vi "Main.vi"() -> ()   [LabVIEW 2026]
doc: "This template is for the Queued Message Handler design pattern.\n\nThe Event Handling Loop generates messages based on user interface actions.\n\nThe Message Handling Loop processes messages generated by the Event Handling Loop, or by other messages. The messages are string values, so new messages can be added easily to the Message Cases case structure in the Message Handling Loop. Each message cluster can also provide an optional value for Message Data, which is a variant that can be converted to whatever message-specific data is required."
uses:
  Controls/Telemetry_Data_Type.ctl
  Controls/Channels.ctl
  Acquisition/Controls/Alarms.ctl
  Controls/UI_Data_Type.ctl
  Controls/Waveforms.ctl
  Controls/UI State.ctl
  Support/Message Queue/Enqueue Message (Single).vi
  <vilib>/Utility/error.llb/Error Cluster From Error Code.vi
  <vilib>/ErrorRing/Error Ring.xnode
  support/Message Queue/Message Queue.lvlib
  support/User Event - Stop/User Event - Stop.lvlib
  Acquisition/Acquisition.lvlib
  TCP/TCP.lvlib
  Database/Database.lvlib
  Data Logging/Data Logging.lvlib
  <vilib>/Analysis/NI_AALPro.lvlib
panel:
  out "Alarms":T1
  out "Telemetry Data":T2
  out "Vibration Frequency Spectrum":waveform(dbl)[](graph)
  out "Vibration Display":waveform(dbl)[](graph)
  in  "Start Acquisition":bool
  out "Display":string
  in  "Exit":bool
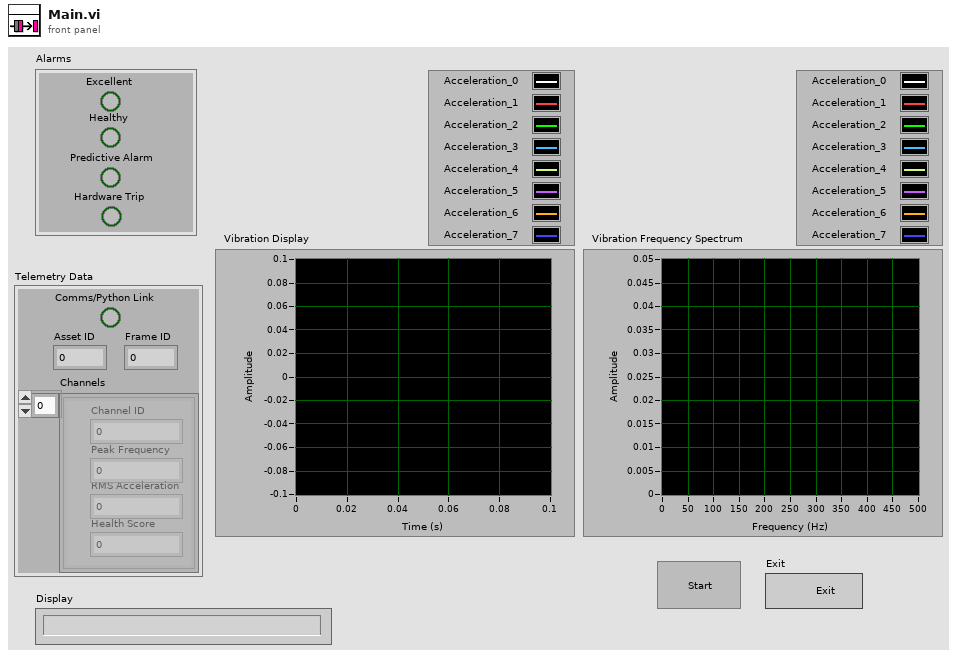
[diagram p1: front panel]
types:
  T1 = typedef "Acquisition.lvlib/Alarms.ctl" = cluster{"Excellent":bool, "Healthy":bool, "Predictive Alarm":bool, "Hardware Trip":bool}
  T2 = typedef "Telemetry_Data_Type.ctl" = cluster{"asset_id":i32, "frame_id":i32, "channels":T3, "comms/python link":bool}
  T3 = typedef "Channels.ctl" = cluster{"channel_id":dbl, "peak_frequency":dbl, "rms_acceleration":dbl, "health_score":dbl}[]
  T4 = typedef "UI State.ctl" = enum16{"Idle", "Acquiring and Logging", "Waiting for Exit", "Waiting for Exit (Acq Stopped)", "Waiting for Exit (Log Stopped)", "Waiting for Stop", "Waiting for Stop (Acq Stopped)", "Waiting for Stop (Log Stopped)"}
  T5 = typedef "Waveforms.ctl" = waveform(dbl)[]
  T6 = typedef "UI_Data_Type.ctl" = cluster{"Boolean":bool, "String":string, "Numeric ":dbl, "Data Display Ref":refnum<vi>, "Exit Button Ref":refnum<vi>}
  T7 = typedef "Message Queue.lvlib/All Message Queues.ctl" = cluster{"UI":refnum<queue>, "Database":refnum<queue>, "TCP":refnum<queue>, "Acquisition":refnum<queue>, "Data Logging":refnum<queue>}
  T8 = typedef "Vibration_Monitor_Config.ctl" = cluster{"Diagnostic_Modes":cluster{"Selected_Mode":string}, "Basic_Health":T9, "Complex_Machinery":T9, "Multi_Point":T9, "System_Settings":T10}
  T9 = typedef "Vibration_Profile.ctl" = cluster{"Task_Name":string, "Sample_Rate_Hz":dbl, "Samples_Per_Channel":i32}
  T10 = typedef "System_Settings.ctl" = cluster{"Simulation_Mode ":string, "Options":T11}
  T11 = typedef "Options.ctl" = enum16{"Healthy", "Unbalance_Alert", "Bearing_Fault_Critical", "Sweep_Test"}
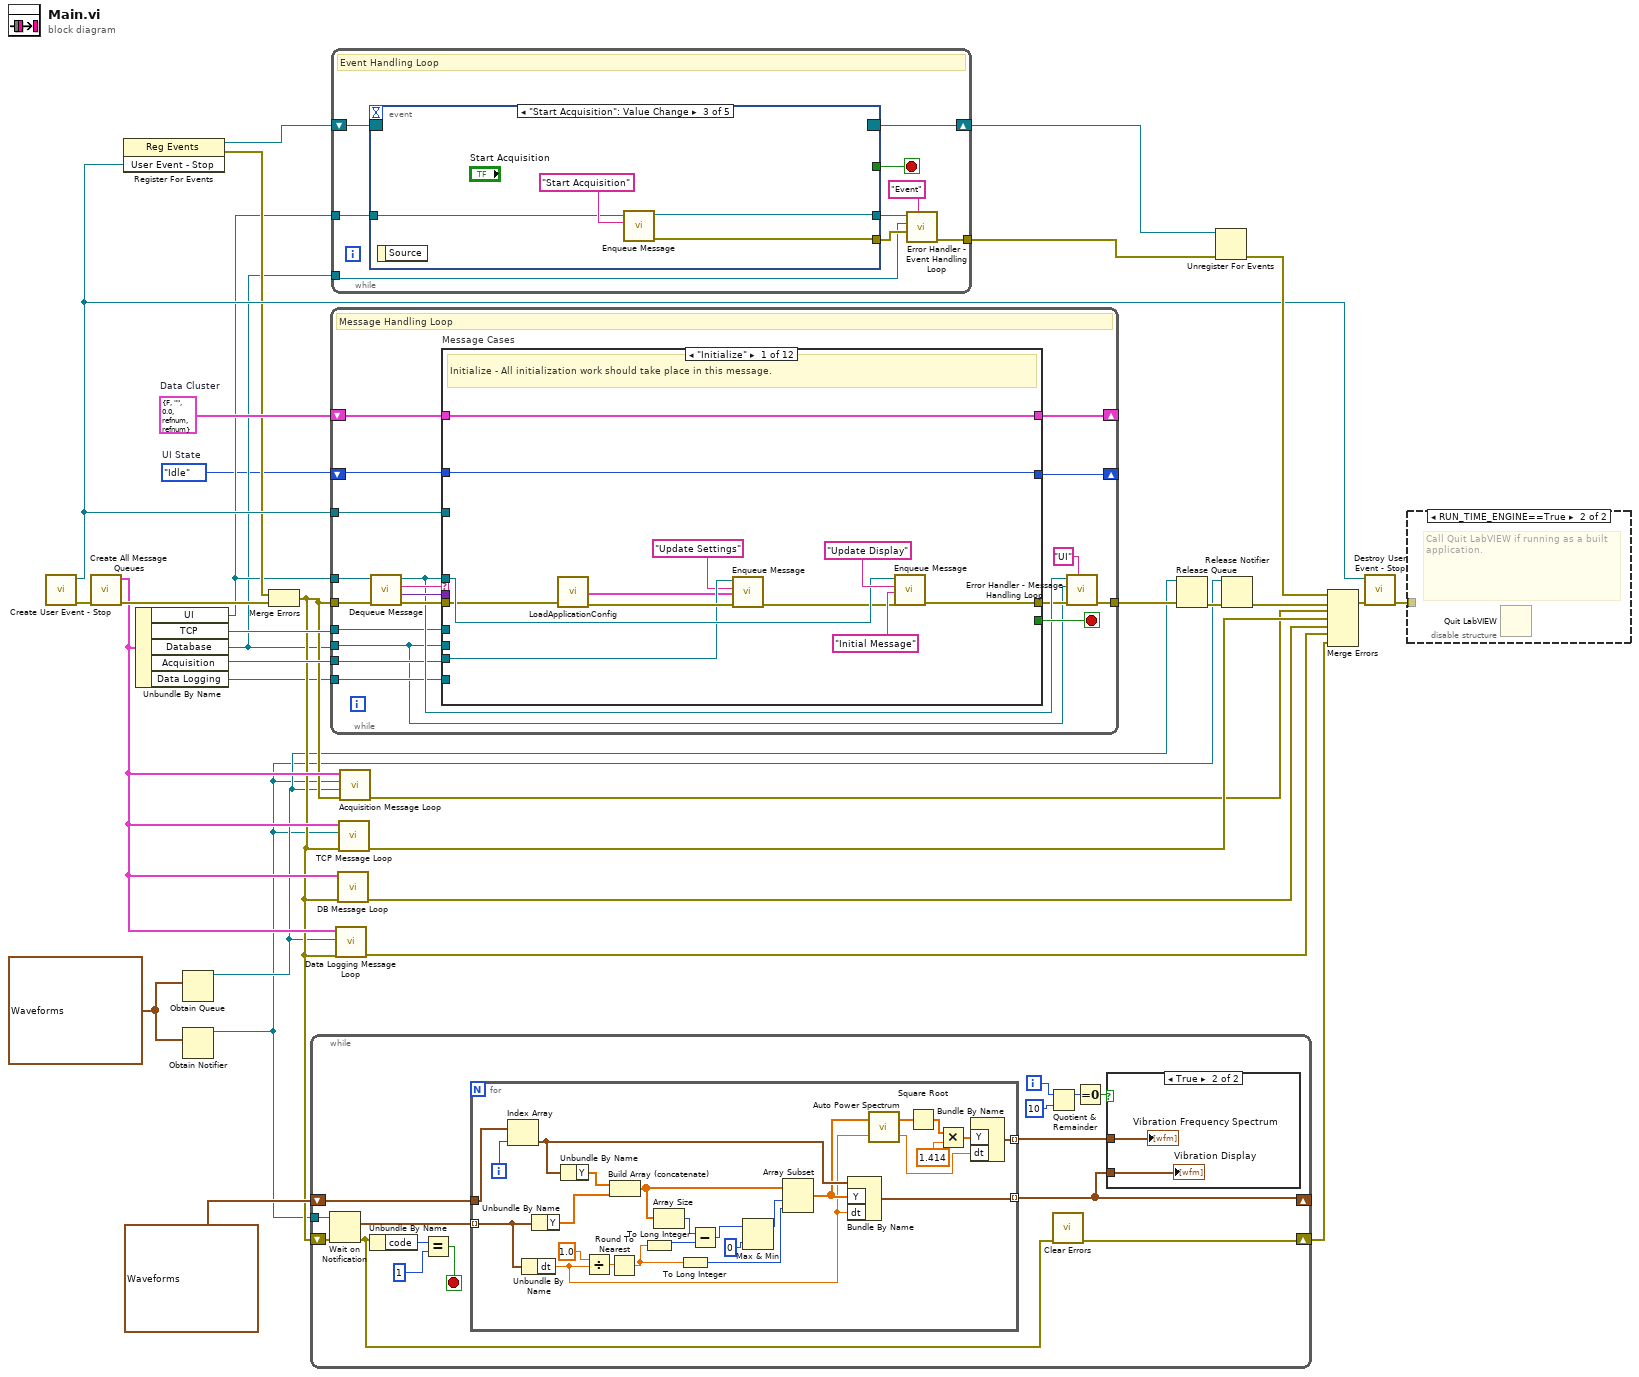
[diagram p0: block diagram]
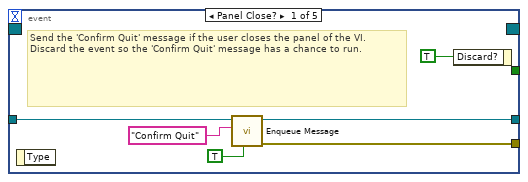
[diagram p4: hidden frame]
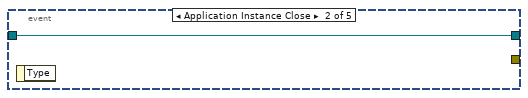
[diagram p5: hidden frame]
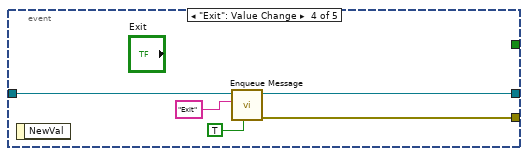
[diagram p6: hidden frame]
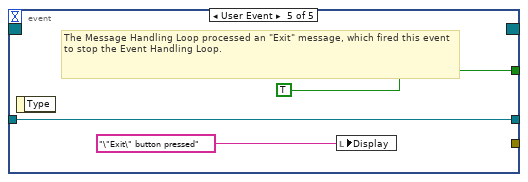
[diagram p7: hidden frame]
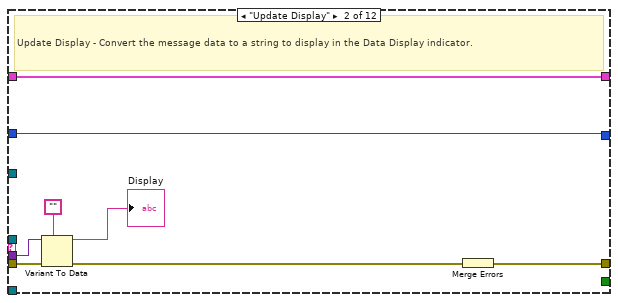
[diagram p8: hidden frame]
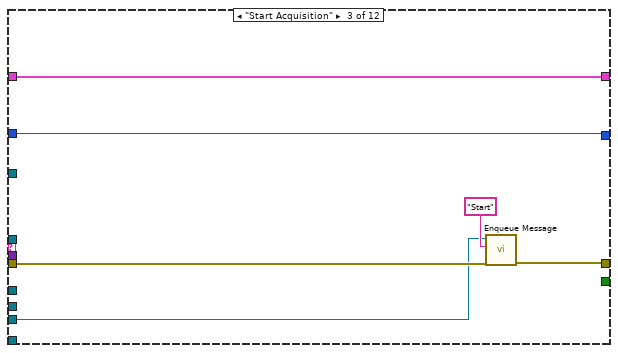
[diagram p9: hidden frame]
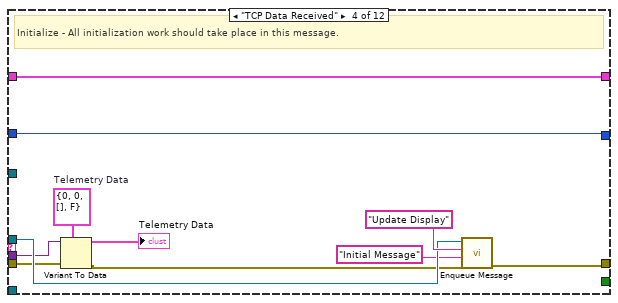
[diagram p10: hidden frame]
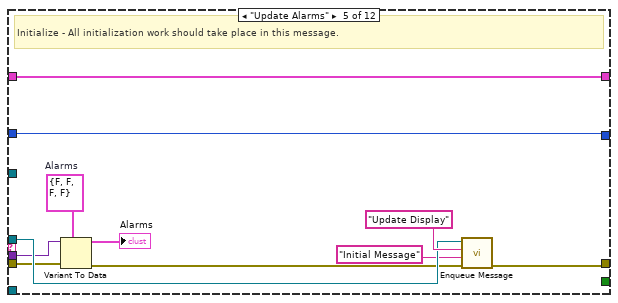
[diagram p11: hidden frame]
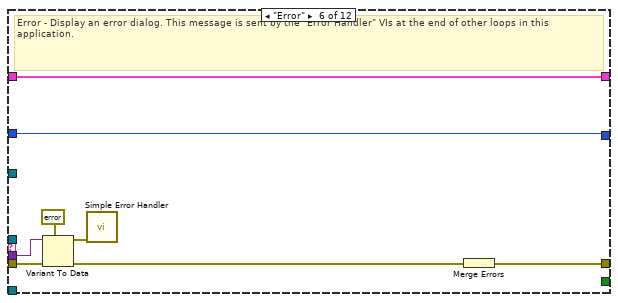
[diagram p12: hidden frame]
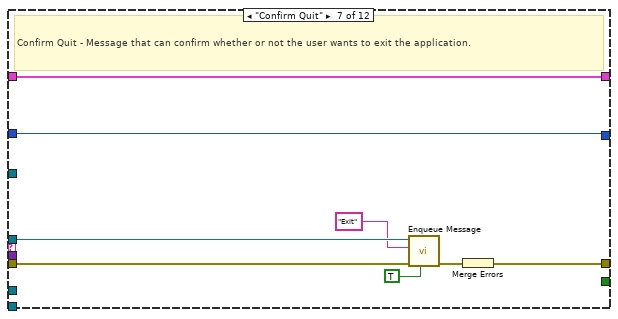
[diagram p13: hidden frame]
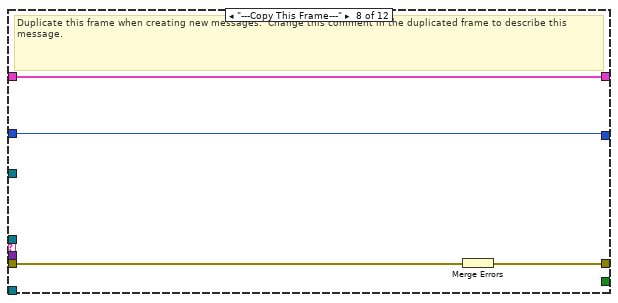
[diagram p14: hidden frame]
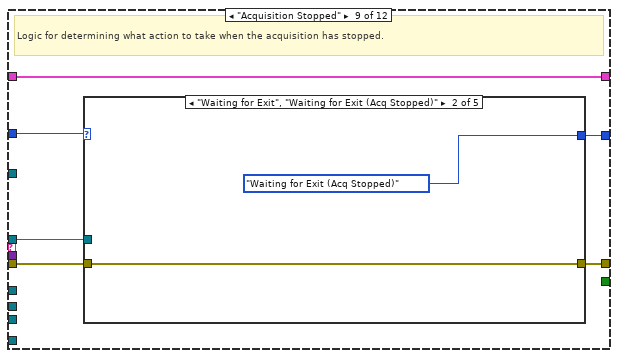
[diagram p15: hidden frame]
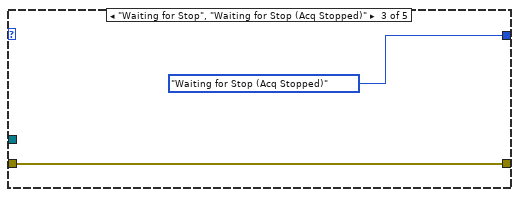
[diagram p17: hidden frame]
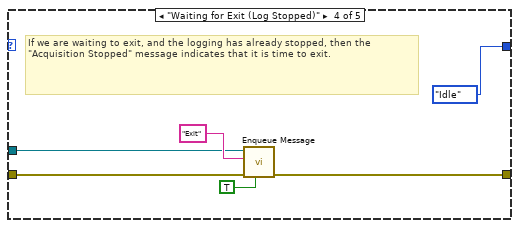
[diagram p18: hidden frame]
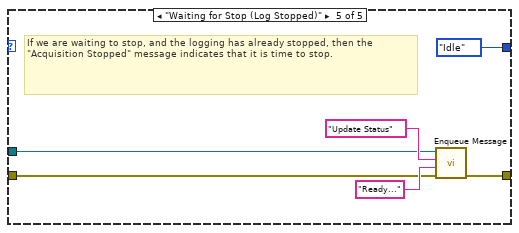
[diagram p19: hidden frame]
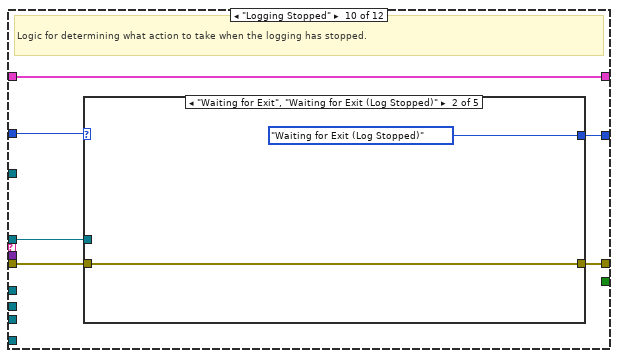
[diagram p20: hidden frame]
diagram:
  w1 = UI_State."Idle"  # UI State
  w17 = T5 [{"t0"=timestamp(0 s since 1904-01-01), "dt"=1.0, "Y"=[0.0]}]
  w26 = T6 {"Boolean"=FALSE, "String"="", "Numeric "=0.0, "Data Display Ref"=refnum, "Exit Button Ref"=refnum}  # Data Cluster
  n1 = call "Create User Event - Stop.vi"() -> ("error out"=w30:errorcluster, "User Event - Stop"=w22:refnum<user-event>)  [unwired: 10 in]
  n2 = call "Create All Message Queues.vi"("error in (no error)"=w30) -> ("error out"=w31:errorcluster, "Message Queues out"=w9:T7)  [unwired: 9 in]
  n3 = register-events(w22) -> (reference out=w23:refnum<event-registration>, error out=w21:errorcluster)  [unwired: 2 in]
  n4 = Unbundle By Name(w9) -> ("UI"=w18:refnum<queue>, "TCP"=w19:refnum<queue>, "Database"=w2:refnum<queue>, "Acquisition"=w11:refnum<queue>, "Data Logging"=w5:refnum<queue>)
  n5 = Obtain Queue(element data type=w17) -> (queue out=w4:refnum<queue>)  [unwired: 4 in, 2 out]
  n6 = Obtain Notifier(notification data type=w17) -> (notifier out=w3:refnum<notifier>)  [unwired: 3 in, 2 out]
  n7 = Merge Errors(w21, w31) -> (w8:errorcluster)
  n8 = while {
    tunnel: w3 -> [w46]
    shift-right: [w39] -> _
    shift-left: T5 [{"t0"=timestamp(0 s since 1904-01-01), "dt"=1.0, "Y"=[0.0]}] ("Waveform") -> [w40]
    shift-right: [w37] -> w7
    shift-left: w8 -> [w45]
    i -> [w36]
    stop <- w44 stop-if-true
    n9 = Wait on Notification(notifier=w46, error in (no error)=w45) -> (notification=w41:T5, error out=w38:errorcluster)  [unwired: 2 in, 2 out]
    n10 = Unbundle By Name(w38) -> ("code"=w43:i32)
    n11 = Equal?(x=w43, y=1) -> (x = y?=w44:bool)
    n12 = for {
      tunnel: w41 -> [w62] mode=indexing
      tunnel: w40 -> [w65]
      tunnel: [w58] -> w39 mode=indexing
      tunnel: [w52] -> w32 mode=indexing
      i -> [w57]
      n13 = Index Array(array=w65, index=w57) -> (element=w63:waveform(dbl))
      n14 = Unbundle By Name(w62) -> ("dt"=w53:dbl)
      n15 = Unbundle By Name(w62) -> ("Y"=w72:dbl[])
      n16 = Unbundle By Name(w63) -> ("Y"=w64:dbl[])
      n17 = Divide(x=1.0, y=w53) -> (x/y=w71:dbl)
      n18 = Round To Nearest(number=w71) -> (nearest integer value=w67:dbl)
      n19 = Build Array (concatenate)(w64, w72) -> (w70:dbl[])
      n20 = To Long Integer(number=w67) -> (32bit integer=w68:i32)
      n21 = Array Size(array=w70) -> (size(s)=w69:i32)
      n22 = To Long Integer(number=w67) -> (32bit integer=w66:i32)
      n23 = Subtract(x=w69, y=w68) -> (x-y=w61:i32)
      n24 = Max & Min(x=w61, y=0) -> (max(x,y)=w59:i32)  [unwired: 1 out]
      n25 = Array Subset(array=w70, index=w59, length=w66) -> (w56:dbl[])
      n26 = Bundle By Name(cluster=w63, "Y"=w56, "dt"=w53) -> (w58:waveform(dbl))
      n27 = call <vilib>:"Auto Power Spectrum.vi"("dt"=w53, "Signal (V)"=w56) -> ("df"=w51:dbl, "Power Spectrum (V^2 rms)"=w50:dbl[])
      n28 = Square Root(x=w50) -> (sqrt(x)=w49:dbl[])
      n29 = Multiply(x=w49, y=1.414) -> (x*y=w54:dbl[])
      n30 = Bundle By Name("Y"=w54, "dt"=w51) -> (w52:waveform(dbl))  [unwired: 1 in]
    }
    n31 = Quotient & Remainder(x=w36, y=10) -> (x-y*floor(x/y)=w34:i32)  [unwired: 1 out]
    n32 = call <vilib>:"Clear Errors.vi"("error in (no error)"=w38) -> ("error out"=w37:errorcluster)  [unwired: 5 in, 1 out]
    n33 = Equal To 0?(x=w34) -> (x = 0?=w33:bool)
    n34 = case shown="True" w33 {
      tunnel: w39 -> [_ w47]
      tunnel: w32 -> [_ w48]
      frame False {
      }
      frame True {
        "Vibration Display" <- w47
        "Vibration Frequency Spectrum" <- w48
      }
    }
  }
  n35 = while {
    tunnel: w18 -> [w84]
    shift-right: [w91] -> _
    shift-left: w26 -> [w92]
    tunnel: w22 -> [w89]
    tunnel: w8 -> [w88]
    tunnel: [w82] -> w15
    tunnel: w19 -> [w80]
    tunnel: w2 -> [w77]
    tunnel: w11 -> [w79]
    tunnel: w5 -> [w78]
    shift-right: [w74] -> _
    shift-left: w1 -> [w75]
    stop <- w90 stop-if-true
    # "Message Handling Loop"
    n36 = call "Dequeue Message.vi"("error in (no error)"=w88, "Message Queue"=w84) -> ("error out"=w87:errorcluster, "Message Data"=w85:variant, "Message"=w86:string, "dup Message Queue"=w83:refnum<queue>)  [unwired: 6 in]
    n37 = case "Message Cases" shown="\"Initialize\"" w86 {
      selector: w86 -> [_ _ _ _ _ _ _ _ _ _ _ w235]
      tunnel: w83 -> [w102 _ _ w127 w138 _ w152 _ w163 w187 w224 _]
      tunnel: w87 -> [w99 w110 w117 w123 w135 w148 w156 w160 w162 w186 w225 _]
      tunnel: [w104 w111 w116 w129 w140 w142 w154 w158 w161 w185 w231 w236] -> w81
      tunnel: w92 -> [w100 w112 w118 w125 w132 w147 w155 w159 w166 w190 w233 w237]
      tunnel: [w100 w112 w118 w125 w132 w147 w155 w159 w166 w190 w233 w237] -> w91
      tunnel: [_ _ _ _ _ _ _ _ _ _ TRUE _] -> w90
      tunnel: w85 -> [_ w109 _ w124 w136 w146 _ _ _ _ w226 _]
      tunnel: w89 -> [_ _ _ _ _ _ _ _ _ _ w230 _]
      tunnel: w80 -> [_ _ _ _ _ _ _ _ _ _ w220 _]
      tunnel: w77 -> [_ _ _ _ _ _ _ _ _ _ w218 _]
      tunnel: w79 -> [w96 _ w114 _ _ _ _ _ _ _ w216 _]
      tunnel: w78 -> [_ _ _ _ _ _ _ _ _ _ w212 _]
      tunnel: w75 -> [w93 w105 w113 w119 w130 w141 w149 w157 w165 w189 w209 w234]
      tunnel: [w93 w105 w113 w119 w130 w141 w149 w157 w164 w188 w209 w234] -> w74
      frame "Initialize" {
        # "Initialize - All initialization work should take place in this message."
        n38 = call "LoadApplicationConfig.vi"("error in (no error)"=w99) -> ("error out"=w98:errorcluster, "Config Cluster"=w94:T8)  [unwired: 8 in, 1 out]
        n39 = call-poly "Enqueue Message.vi"("error in (no error)"=w98, "Message Data"=w94, "Message"="Update Settings", "Message Queue"=w96) -> ("error out"=w97:errorcluster)  [unwired: 6 in, 1 out]
        n40 = call-poly "Enqueue Message.vi"("error in (no error)"=w97, "Message Data"="Initial Message" ("Initial Message"), "Message"="Update Display", "Message Queue"=w102) -> ("error out"=w104:errorcluster)  [unwired: 6 in, 1 out]
      }
      frame "Update Display" {
        # "Update Display - Convert the message data to a string to display in the Data Display indicator."
        n41 = Variant To Data(error in=w110, type="", Variant=w109) -> (data=→"Display":string, error out=w107:errorcluster)
        n42 = Merge Errors(w107) -> (w111:errorcluster)
      }
      frame "Start Acquisition" {
        n43 = call-poly "Enqueue Message.vi"("error in (no error)"=w117, "Message"="Start", "Message Queue"=w114) -> ("error out"=w116:errorcluster)  [unwired: 7 in, 1 out]
      }
      frame "TCP Data Received" {
        w122 = T2 {"asset_id"=0, "frame_id"=0, "channels"=[], "comms/python link"=FALSE}  # Telemetry Data
        # "Initialize - All initialization work should take place in this message."
        n44 = Variant To Data(error in=w123, type=w122, Variant=w124) -> (data=→"Telemetry Data":T2, error out=w121:errorcluster)
        n45 = call-poly "Enqueue Message.vi"("error in (no error)"=w121, "Message Data"="Initial Message" ("Initial Message"), "Message"="Update Display", "Message Queue"=w127) -> ("error out"=w129:errorcluster)  [unwired: 6 in, 1 out]
      }
      frame "Update Alarms" {
        w133 = T1 {"Excellent"=FALSE, "Healthy"=FALSE, "Predictive Alarm"=FALSE, "Hardware Trip"=FALSE}  # Alarms
        # "Initialize - All initialization work should take place in this message."
        n46 = Variant To Data(error in=w135, type=w133, Variant=w136) -> (data=→"Alarms":T1, error out=w134:errorcluster)
        n47 = call-poly "Enqueue Message.vi"("error in (no error)"=w134, "Message Data"="Initial Message" ("Initial Message"), "Message"="Update Display", "Message Queue"=w138) -> ("error out"=w140:errorcluster)  [unwired: 6 in, 1 out]
      }
      frame "Error" {
        # "Error - Display an error dialog. This message is sent by the \"Error Handler\" VIs at the end of other loops in this application."
        n48 = Variant To Data(error in=w148, type=errorcluster {"status"=FALSE, "code"=0, "source"=""} ("error constant"), Variant=w146) -> (data=w144:errorcluster, error out=w143:errorcluster)
        n49 = call <vilib>:"Simple Error Handler.vi"("error in (no error)"=w144) -> ()  [unwired: 4 in, 5 out]
        n50 = Merge Errors(w143) -> (w142:errorcluster)
      }
      frame "Confirm Quit" {
        # "Confirm Quit - Message that can confirm whether or not the user wants to exit the application."
        n51 = call-poly "Enqueue Message.vi"("Priority Message? (F)"=TRUE, "error in (no error)"=w156, "Message"="Exit", "Message Queue"=w152) -> ("error out"=w153:errorcluster)  [unwired: 6 in, 1 out]
        n52 = Merge Errors(w153) -> (w154:errorcluster)
      }
      frame "---Copy This Frame---" {
        # "Duplicate this frame when creating new messages.  Change this comment in the duplicated frame to describe this message."
        n53 = Merge Errors(w160) -> (w158:errorcluster)
      }
      frame "Acquisition Stopped" {
        # "Logic for determining what action to take when the acquisition has stopped."
        n54 = case shown="\"Waiting for Exit\", \"Waiting for Exit (Acq Stopped)\"" w165 {
          selector: w165 -> [w168 _ _ _ _]
          tunnel: [w168 UI_State."Waiting for Exit (Acq Stopped)" ("UI State") UI_State."Waiting for Stop (Acq Stopped)" ("UI State") UI_State."Idle" ("UI State") UI_State."Idle" ("UI State")] -> w164
          tunnel: [w167 w169 w171 w178 w183] -> w161
          tunnel: w163 -> [_ _ _ w174 w180]
          tunnel: w162 -> [w167 w169 w171 w173 w179]
          frame Default {
          }
          frame "Waiting for Exit", "Waiting for Exit (Acq Stopped)" {
          }
          frame "Waiting for Stop", "Waiting for Stop (Acq Stopped)" {
          }
          frame "Waiting for Exit (Log Stopped)" {
            # "If we are waiting to exit, and the logging has already stopped, then the \"Acquisition Stopped\" message indicates that it is time to exit."
            n55 = call-poly "Enqueue Message.vi"("Priority Message? (F)"=TRUE, "error in (no error)"=w173, "Message"="Exit", "Message Queue"=w174) -> ("error out"=w178:errorcluster)  [unwired: 6 in, 1 out]
          }
          frame "Waiting for Stop (Log Stopped)" {
            # "If we are waiting to stop, and the logging has already stopped, then the \"Acquisition Stopped\" message indicates that it is time to stop."
            n56 = call-poly "Enqueue Message.vi"("error in (no error)"=w179, "Message Data"="Ready..." ("Ready..."), "Message"="Update Status", "Message Queue"=w180) -> ("error out"=w183:errorcluster)  [unwired: 6 in, 1 out]
          }
        }
      }
      frame "Logging Stopped" {
        # "Logic for determining what action to take when the logging has stopped."
        n57 = case shown="\"Waiting for Exit\", \"Waiting for Exit (Log Stopped)\"" w189 {
          selector: w189 -> [w192 _ _ _ _]
          tunnel: [w192 UI_State."Waiting for Exit (Log Stopped)" ("UI State") UI_State."Waiting for Stop (Log Stopped)" ("UI State") UI_State."Idle" ("UI State") UI_State."Idle" ("UI State")] -> w188
          tunnel: [w191 w193 w195 w202 w207] -> w185
          tunnel: w187 -> [_ _ _ w198 w204]
          tunnel: w186 -> [w191 w193 w195 w197 w203]
          frame Default {
          }
          frame "Waiting for Exit", "Waiting for Exit (Log Stopped)" {
          }
          frame "Waiting for Stop", "Waiting for Stop (Log Stopped)" {
          }
          frame "Waiting for Exit (Acq Stopped)" {
            # "If we are waiting to exit, and the acquisition has already stopped, then the \"Logging Stopped\" message indicates that it is time to exit."
            n58 = call-poly "Enqueue Message.vi"("Priority Message? (F)"=TRUE, "error in (no error)"=w197, "Message"="Exit", "Message Queue"=w198) -> ("error out"=w202:errorcluster)  [unwired: 6 in, 1 out]
          }
          frame "Waiting for Stop (Acq Stopped)" {
            # "If we are waiting to stop, and the acquisition has already stopped, then the \"Logging Stopped\" message indicates that it is time to stop."
            n59 = call-poly "Enqueue Message.vi"("error in (no error)"=w203, "Message Data"="Ready..." ("Ready..."), "Message"="Update Status", "Message Queue"=w204) -> ("error out"=w207:errorcluster)  [unwired: 6 in, 1 out]
          }
        }
      }
      frame "Exit" {
        # "Stop the VI"
        # "Release the message queue reference"
        # "Exit - Exit the application."
        n60 = Variant To Data(type=errorcluster {"status"=FALSE, "code"=0, "source"=""} ("error constant"), Variant=w226) -> (data=w227:errorcluster)  [unwired: 1 in, 1 out]
        n61 = call <vilib>:"Simple Error Handler.vi"("error in (no error)"=w227) -> ()  [unwired: 4 in, 5 out]
        n62 = call-poly "Enqueue Message.vi"("error in (no error)"=w225, "Message"="Exit", "Message Queue"=w218) -> ("error out"=w221:errorcluster)  [unwired: 7 in, 1 out]
        n63 = call-poly "Enqueue Message.vi"("Priority Message? (F)"=TRUE, "error in (no error)"=w221, "Message"="Exit", "Message Queue"=w220) -> ("error out"=w215:errorcluster)  [unwired: 6 in, 1 out]
        n64 = call-poly "Enqueue Message.vi"("error in (no error)"=w215, "Message"="Exit", "Message Queue"=w216) -> ("error out"=w211:errorcluster)  [unwired: 7 in, 1 out]
        n65 = call-poly "Enqueue Message.vi"("error in (no error)"=w211, "Message"="Exit", "Message Queue"=w212) -> ("error out"=w214:errorcluster)  [unwired: 7 in, 1 out]
        n66 = call "Fire User Event - Stop.vi"("User Event - Stop"=w230) -> ("error out"=w229:errorcluster)  [unwired: 10 in]
        n67 = Release Queue(queue=w224, error in (no error)=w214) -> (error out=w219:errorcluster)  [unwired: 1 in, 2 out]
        n68 = Merge Errors(w229, w219) -> (w231:errorcluster)
      }
      frame Default {
        # "'Default' case only runs if there is a message that isn't defined in any of the other cases.  Output a programming error."
        n69 = xnode "Error Ring"("parameter 0"=w235) -> ("error out"=w236:errorcluster)
      }
    }
    n70 = call "Error Handler - Message Handling Loop.vi"("Loop Name"="UI", "error in (no error)"=w81, "Database"=w77, "Message Queue"=w83) -> ("dup error in"=w82:errorcluster)  [unwired: 6 in, 1 out]
  }
  n71 = while {
    tunnel: w18 -> [w253]
    shift-right: [w251] -> w27
    shift-left: w23 -> [w252]
    tunnel: [w248] -> w24
    tunnel: w2 -> [w245]
    stop <- w250 stop-if-true
    # "Event Handling Loop"
    n72 = event shown="[2] \"Start Acquisition\": Value Change" {
      selector: w252 -> [_ _ _ _ _]
      dyn-events: [_ _ _ _ _] -> w251
      timeout: _ -> [_ _ _ _ _]
      tunnel: [_ _ _ _ TRUE ("Discard?")] -> w250
      tunnel: w253 -> [w258 w260 w263 w269 w272]
      tunnel: [w257 _ w261 w268 _] -> w247
      tunnel: [w256 w260 w262 w267 w272] -> w249
      event Panel Close? {
        # "Send the 'Confirm Quit' message if the user closes the panel of the VI. Discard the event so the 'Confirm Quit' message has a chance to run."
        n73 = event-data() -> ()  [unwired: 1 in, 1 out]
        n74 = call-poly "Enqueue Message.vi"("Priority Message? (F)"=TRUE, "Message"="Confirm Quit", "Message Queue"=w258) -> ("error out"=w257:errorcluster, "dup Message Queue"=w256:refnum<queue>)  [unwired: 7 in]
        n75 = event-data("Discard?"=TRUE) -> ()  [unwired: 1 in, 1 out]
      }
      event Application Instance Close {
        n76 = event-data() -> ()  [unwired: 1 in, 1 out]
      }
      event "Start Acquisition": Value Change {
        n77 = event-data() -> ()  [unwired: 1 in, 1 out]
        n78 = call-poly "Enqueue Message.vi"("Message"="Start Acquisition", "Message Queue"=w263) -> ("error out"=w261:errorcluster, "dup Message Queue"=w262:refnum<queue>)  [unwired: 8 in]
      }
      event "Exit": Value Change {
        n79 = event-data() -> ()  [unwired: 1 in, 1 out]
        n80 = call-poly "Enqueue Message.vi"("Priority Message? (F)"=TRUE, "Message"="Exit", "Message Queue"=w269) -> ("error out"=w268:errorcluster, "dup Message Queue"=w267:refnum<queue>)  [unwired: 7 in]
      }
      event User Event {
        # "The Message Handling Loop processed an \"Exit\" message, which fired this event to stop the Event Handling Loop."
        n81 = event-data() -> ()  [unwired: 1 in, 1 out]
        n82 = local write "Display"("\"Exit\" button pressed" ("VI Stopped")) -> ()
      }
    }
    n83 = call "Error Handler - Event Handling Loop.vi"("Loop"="Event", "error in (no error)"=w247, "Database"=w245, "Message Queue"=w249) -> ("dup error in"=w248:errorcluster)  [unwired: 6 in, 1 out]
  }
  n84 = call "Data Logging Message Loop.vi"("error in (no error)"=w8, "Data Queue"=w4, "Message Queues"=w9) -> ("error out"=w6:errorcluster)  [unwired: 8 in]
  n85 = call "DB Message Loop.vi"("error in (no error)"=w8, "Message Queues"=w9) -> ("error out"=w20:errorcluster)  [unwired: 9 in]
  n86 = call "TCP Message Loop.vi"("error in (no error)"=w8, "Data Notifier"=w3, "Message Queues"=w9) -> ("error out"=w13:errorcluster)  [unwired: 8 in]
  n87 = call "Acquisition Message Loop.vi"("error in (no error)"=w8, "Data Queue"=w4, "Data Notifier"=w3, "Message Queues"=w9) -> ("error out"=w12:errorcluster)  [unwired: 7 in]
  n88 = Release Queue(queue=w4, error in (no error)=w15) -> (error out=w16:errorcluster)  [unwired: 1 in, 2 out]
  n89 = Unregister For Events(event registration refnum=w27, error in=w24) -> (error out=w28:errorcluster)
  n90 = Release Notifier(notifier=w3, error in (no error)=w16) -> (error out=w14:errorcluster)  [unwired: 1 in, 2 out]
  n91 = Merge Errors(w28, w14, w12, w13, w20, w6, w7) -> (w29:errorcluster)
  n92 = call "Destroy User Event - Stop.vi"("error in (no error)"=w29, "User Event - Stop"=w22) -> ("error out"=w25:errorcluster)  [unwired: 9 in]
  n93 = disable-structure shown="RUN_TIME_ENGINE==True" {
    disable-tunnel: w25 -> [_ _]
    frame condition #0 (active) {
    }
    frame condition #1 {
      # "Call Quit LabVIEW if running as a built application."
      n94 = Quit LabVIEW() -> ()  [unwired: 1 in]
    }
  }
